vi "Sine Out.vi"() -> ()   [LabVIEW 2020]
uses:
  Submodules/Source/Types/Sine.Generate.Settings.ctl
  <vilib>/rvi/Emulation/niFpgaGetClockAttributes.vi
  <vilib>/rvi/Emulation/niFpgaSctlEmulationGetInTimedLoop.vi
  <vilib>/rvi/Emulation/niFpgaEmulationReportErrorSimple.vi
  <vilib>/rvi/Emulation/niFpgaCriticalErrorInLSC.vi
  Submodules/Source/Speciality FPGA IO.lvlib
panel:
  out "PERIODS/TICKS":fxp<+,32,0>
  out "OFFSET":fxp<+/-,32,8>
  out "AMP":fxp<+/-,32,8>
  in  "Sine Out":T1
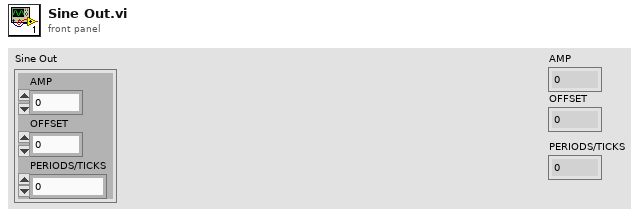
[diagram p1: front panel]
types:
  T1 = typedef "Speciality FPGA IO.lvlib/Sine.Generate.Settings.ctl" = cluster{"AMP":fxp<+/-,32,8>, "OFFSET":fxp<+/-,32,8>, "PERIODS/TICKS":fxp<+,32,0>}
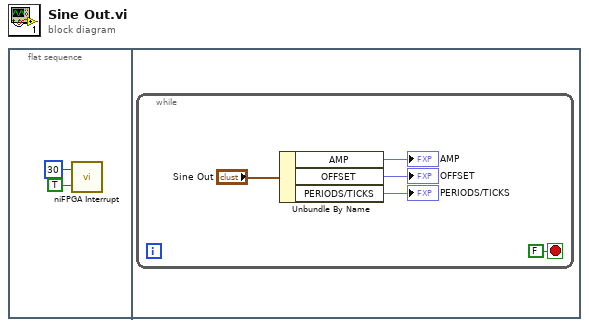
[diagram p0: block diagram]
diagram:
  n1 = flat-sequence {
    frame #0 {
      n2 = call <vilib>:"niFPGA Interrupt.vi"("Wait Until Cleared (F)"=TRUE, "IRQ Number (0)"=u8 30) -> ()  [unwired: 1 in]
    }
    frame #1 {
      n3 = while {
        stop <- FALSE stop-if-true
        n4 = Unbundle By Name("Sine Out") -> ("AMP"=→"AMP":fxp<+/-,32,8>, "OFFSET"=→"OFFSET":fxp<+/-,32,8>, "PERIODS/TICKS"=→"PERIODS/TICKS":fxp<+,32,0>)
      }
    }
  }
